vi "find_interference_len.vi"(8 "干涉长度":i32=50, 9 "阈值":dbl=2.2, 10 "A":dbl[](array[numeric])=array[267857 elements], 11 "S":dbl[](array[numeric])=array[267857 elements]) -> (1 "Max_Index":i32, 2 "个数":u32=2, 3 "INDEX":i32[](array[numeric]))   [LabVIEW 2015, in "Boimetry Processing.lvlib"]
uses:
  Boimetry Processing.lvlib
  <vilib>/Analysis/NI_AALPro.lvlib
  <vilib>/Analysis/NI_AAL_SigProc.lvlib
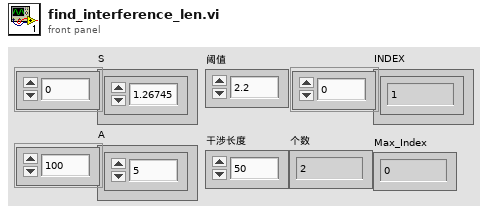
[diagram p1: front panel]
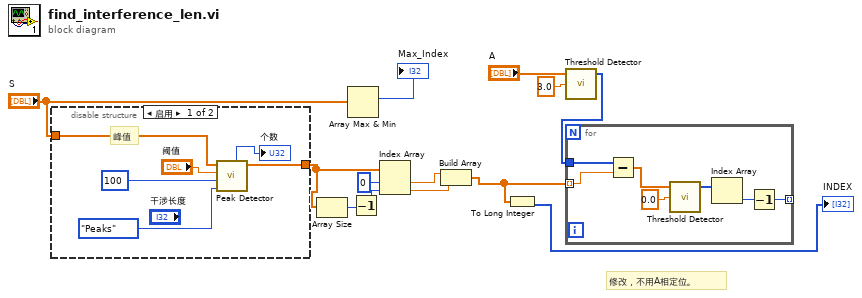
[diagram p0: block diagram]
diagram:
  # "修改，不用A相定位。"
  n1 = disable-structure shown="启用" {
    disable-tunnel: "S" -> [w19 _]
    disable-tunnel: [w15 _] -> w8
    frame Enabled {
      # "峰值"
      n2 = call <vilib>:"Peak Detector.vi"("peaks/valleys"=enum32{"Peaks", "Valleys"}."Peaks", "width"=100, "threshold"="阈值", "X"=w19) -> ("Locations"=w15:dbl[], "# found"=→"个数":i32)  [unwired: 3 in, 3 out]
    }
    frame Disabled {
    }
  }
  n3 = Array Size(array=w8) -> (size(s)=w7:i32)
  n4 = Array Max & Min(array="S") -> (max index (indices)=→"Max_Index":i32)  [unwired: 3 out]
  n5 = Decrement(x=w7) -> (x-1=w6:i32)
  n6 = Index Array(array=w8, index #1=0 ("索引"), index #2=w6) -> (element #1=w4:dbl, element #2=w3:dbl)
  n7 = Build Array(w4, w3) -> (w2:dbl[])
  n8 = To Long Integer(number=w2) -> (32bit integer=→"INDEX":i32[])
  n9 = call <vilib>:"Threshold Detector.vi"("threshold"=3.0, "X"="A") -> ("Indices"=w10:i32[])  [unwired: 1 in, 2 out]
  n10 = for {
    tunnel: w2 -> [w26] mode=indexing
    tunnel: w10 -> [w22]
    tunnel: [w20] -> _ mode=indexing
    n11 = Subtract(x=w22, y=w26) -> (x-y=w24:dbl[])
    n12 = call <vilib>:"Threshold Detector.vi"("threshold"=0.0, "X"=w24) -> ("Indices"=w23:i32[])  [unwired: 1 in, 2 out]
    n13 = Index Array(array=w23) -> (element=w21:i32)  [unwired: 1 in]
    n14 = Decrement(x=w21) -> (x-1=w20:i32)
  }
